vi "FITS_WriteGeomSingle.vi"(0 "amplifier":string, 1 "Tsec":string, 2 "file ref":u64, 3 "Dsec":string, 4 "Csec":string, 5 "Bsec":string, 6 "Asec":string) -> ()   [LabVIEW 2016]
uses:
  usr/local/lib/libfits.so
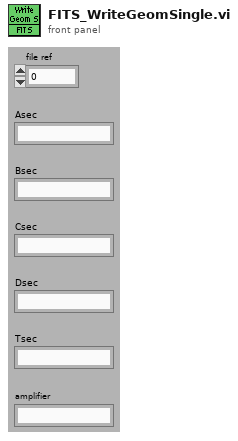
[diagram p1: front panel]
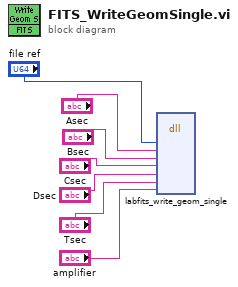
[diagram p0: block diagram]
diagram:
  n1 = dll-call lib="usr/local/lib/libfits.so" fn="labfits_write_geom_single"("ref"="file ref", "Asec"="Asec", "Bsec"="Bsec", "Csec"="Csec", "Dsec"="Dsec", "Tsec"="Tsec", "amplifier"="amplifier") -> ()  [unwired: 10 in, 3 out]
